vi "Cal1-GetPath.vi"(8 "Mode in":T1, 11 "Calib file":path) -> (1 "String output":string, 2 "exists?":bool, 3 "Path output":path)   [LabVIEW 2018]
uses:
  Anemometry Sub Vis/Calibration/Calib_mode.ctl
  Anemometry Sub Vis/Globals/Calib_global.vi
  Anemometry Sub Vis/Globals/Meas_global.vi
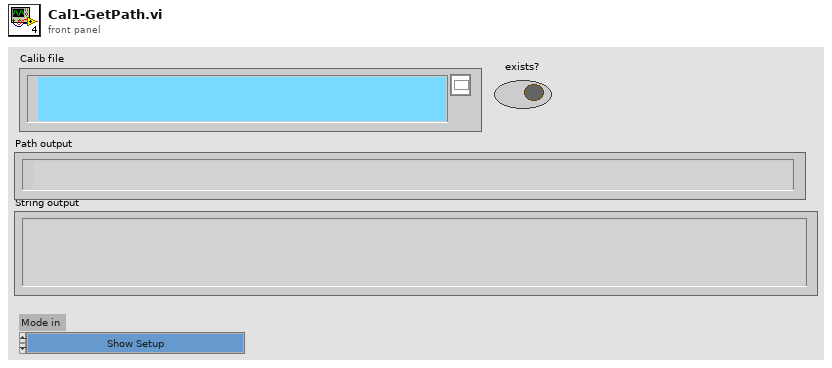
[diagram p1: front panel]
types:
  T1 = typedef "Calib_mode.ctl" = enum16{"Show Setup", "Take a New Calibration Point", "Refit Curve", "Setup Front Panel"}
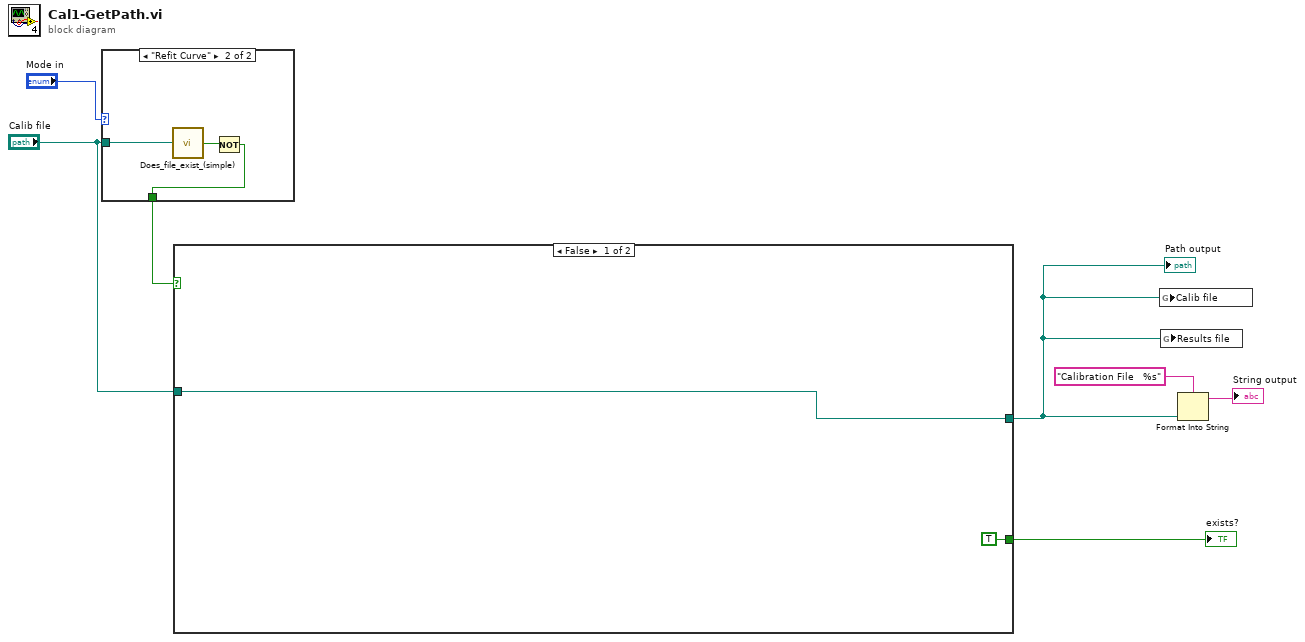
[diagram p0: block diagram]
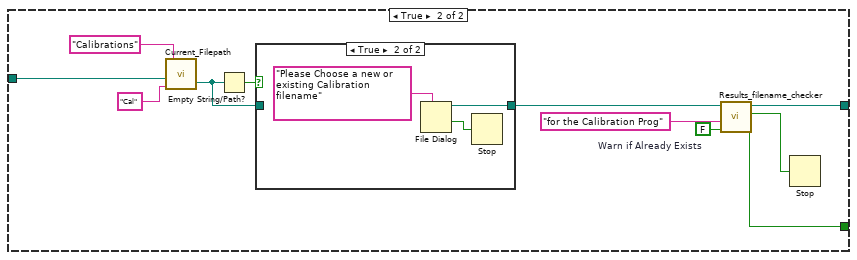
[diagram p2: hidden frame]
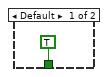
[diagram p4: hidden frame]
diagram:
  n1 = case shown="\"Refit Curve\"" "Mode in" {
    tunnel: "Calib file" -> [_ w11]
    tunnel: [TRUE w9] -> w1
    frame Default {
    }
    frame "Refit Curve" {
      n2 = call "Does_file_exist_(simple).vi"("Pathname"=w11) -> ("exists?"=w10:bool)
      n3 = Not(x=w10) -> (.not. x?=w9:bool)
    }
  }
  n4 = case shown="False" w1 {
    tunnel: [w13 w21] -> w6
    tunnel: [TRUE ("exists?") w17] -> w4
    tunnel: "Calib file" -> [w13 w14]
    frame False {
    }
    frame True {
      w16 = FALSE  # Warn if Already Exists
      n5 = call "Current_Filepath.vi"("Short_Name"="Cal" ("Data Type"), "Filename in"=w14, "Data Type"="Calibrations") -> ("Filename Out"=w22:path)  [unwired: 1 in, 1 out]
      n6 = Empty String/Path?(string/path=w22) -> (empty?=w20:bool)
      n7 = case shown="True" w20 {
        tunnel: w22 -> [w25 _]
        tunnel: [w25 w27] -> w18
        frame False {
        }
        frame True {
          n8 = File Dialog(7:"Please Choose a new or existing Calibration filename" ("Promp if not found")) -> (1:w26:bool, 3:w27:path)  [unwired: 1 in, 7 out]
          n9 = Stop(stop? (T)=w26) -> ()
        }
      }
      n10 = call "Results_filename_checker.vi"("Warn if Already Exists"=w16, "Comment"="for the Calibration Prog", "Results file"=w18) -> ("exists?"=w17:bool, "cancelled"=w19:bool, "Results file output"=w21:path)  [unwired: 1 in, 2 out]
      n11 = Stop(stop? (T)=w19) -> ()
    }
  }
  "Path output" <- w6
  "exists?" <- w4
  n12 = global write "Calib_global.vi" "Calib file"(w6) -> ()
  n13 = global write "Meas_global.vi" "Results file"(w6) -> ()
  n14 = Format Into String(format string="Calibration File   %s", w6) -> (resulting string=→"String output":string)  [unwired: 2 in, 1 out]
